vi "查询员工.vi"(8 "error in (no error)":errorcluster, 11 "员工ID":string="ZJWABY0001") -> (0 "error out":errorcluster, 1 "权限":string, 2 "姓名":string, 3 "索引结果":bool)   [LabVIEW 2013]
uses:
  <vilib>/Utility/error.llb/whitespace.ctl
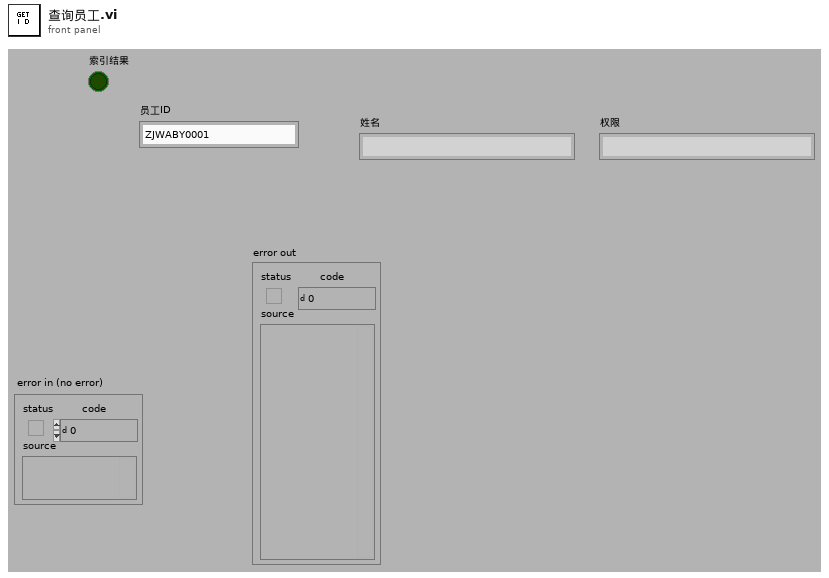
[diagram p1: front panel]
types:
  T1 = typedef "whitespace.ctl" = u16
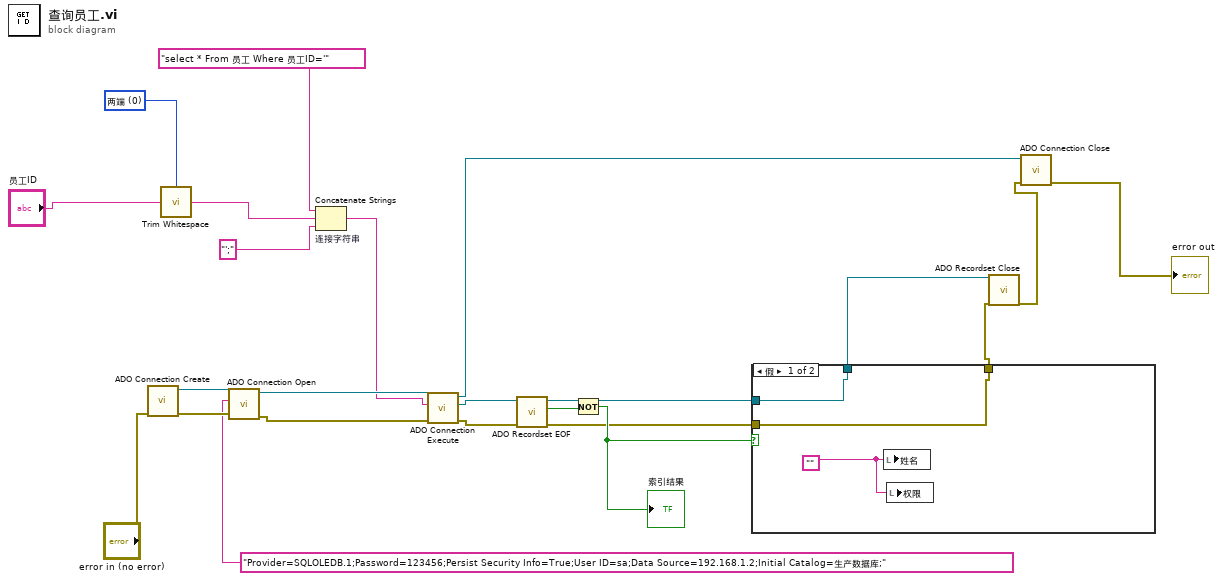
[diagram p0: block diagram]
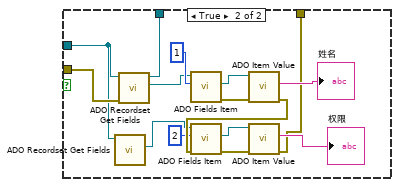
[diagram p2: hidden frame]
diagram:
  w11 = T1 0 items=["两端", "字符串首端", "字符串末端"] ("location (both)")
  n1 = call "ADO Connection Create.vi"("error in (no error)"="error in (no error)") -> ("error out"=w22:errorcluster, "ADODB._Connection Out"=w23:refnum<k7>)  [unwired: 9 out]
  n2 = call <vilib>:"Trim Whitespace.vi"("string"="员工ID", "location (both)"=w11) -> ("trimmed string"=w12:string)
  n3 = call "ADO Connection Open.vi"("error in (no error)"=w22, "ConnectionString"="Provider=SQLOLEDB.1;Password=123456;Persist Security Info=True;User ID=sa;Data Source=192.168.1.2;Initial Catalog=生产数据库;" ("字符串 2"), "ADODB._Connection In"=w23) -> ("error out"=w21:errorcluster, "ADODB._Connection Out"=w20:refnum<k7>)  [unwired: 7 out]
  n4 = Concatenate Strings "连接字符串"("select * From 员工 Where 员工ID='" ("字符串 2"), w12, "';" ("字符串 2")) -> (w10:string)
  n5 = call "ADO Connection Execute.vi"("error in (no error)"=w21, "CommandText"=w10, "ADODB._Connection In"=w20) -> ("error out"=w18:errorcluster, "RecordSet"=w1:refnum<k7>, "ADODB._Connection Out"=w15:refnum<k7>)  [unwired: 6 out]
  n6 = call "ADO Recordset EOF.vi"("error in (no error)"=w18, "ADODB._Recordset In"=w1) -> ("error out"=w5:errorcluster, "EOF"=w17:bool, "ADODB._Recordset Out"=w6:refnum<k7>)  [unwired: 7 out]
  n7 = Not(x=w17) -> (.not. x?=w7:bool)
  "索引结果" <- w7
  n8 = case shown="假" w7 {
    tunnel: w6 -> [w25 w27]
    tunnel: w5 -> [w26 w41]
    tunnel: [w25 w40] -> w4
    tunnel: [w26 w30] -> w3
    frame False {
      w24 = ""
      n9 = local write "姓名"(w24) -> ()
      n10 = local write "权限"(w24) -> ()
    }
    frame True {
      n11 = call "ADO Recordset Get Fields.vi"("ADODB._Recordset In"=w27) -> ("Fields Out"=w29:refnum<k7>)  [unwired: 1 in, 9 out]
      n12 = call "ADO Recordset Get Fields.vi"("error in (no error)"=w41, "ADODB._Recordset In"=w27) -> ("Fields Out"=w33:refnum<k7>, "ADODB._Recordset Out"=w40:refnum<k7>)  [unwired: 8 out]
      n13 = call "ADO Fields Item.vi"("Index"=1, "Fields In"=w33) -> ("error out"=w38:errorcluster, "Item Out"=w37:refnum<k7>)  [unwired: 1 in, 7 out]
      n14 = call "ADO Item Value.vi"("error in (no error)"=w38, "Item In"=w37) -> ("error out"=w34:errorcluster, "Value"=→"姓名":string)  [unwired: 8 out]
      n15 = call "ADO Fields Item.vi"("error in (no error)"=w34, "Index"=2, "Fields In"=w29) -> ("error out"=w35:errorcluster, "Item Out"=w28:refnum<k7>)  [unwired: 7 out]
      n16 = call "ADO Item Value.vi"("error in (no error)"=w35, "Item In"=w28) -> ("error out"=w30:errorcluster, "Value"=→"权限":string)  [unwired: 8 out]
    }
  }
  n17 = call "ADO Recordset Close.vi"("ADODB._Recordset In"=w4, "error in (no error)"=w3) -> ("error out"=w16:errorcluster)  [unwired: 17 out]
  n18 = call "ADO Connection Close.vi"("error in (no error)"=w16, "ADODB._Connection In"=w15) -> ("error out"=→"error out":errorcluster)  [unwired: 9 out]
